vi "Coincident panel edges test.vi"(1 "epsilon":sgl, 3 "V1_1":sgl[](array[numeric])=[1.0, 0.0, 0.0], 4 "V1_0":sgl[](array[numeric])=[1.0, 0.0, 0.0], 5 "V0_1":sgl[](array[numeric])=[1.0, 0.0, 0.0], 6 "V0_0":sgl[](array[numeric])=[1.0, 0.0, 0.0]) -> (0 "Edges are coincident":bool)   [LabVIEW 2017]
panel:
  # "PN 23/10/17"
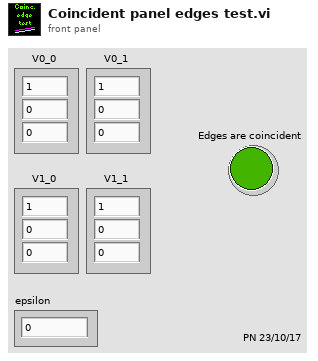
[diagram p1: front panel]
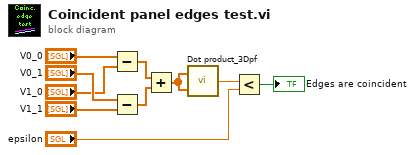
[diagram p0: block diagram]
diagram:
  n1 = Subtract(x="V0_0", y="V1_0") -> (x-y=w10:sgl[])
  n2 = Subtract(x="V0_1", y="V1_1") -> (x-y=w9:sgl[])
  n3 = Add(x=w10, y=w9) -> (x+y=w8:sgl[])
  n4 = call "Dot product_3Dpf.vi"("B"=w8, "A"=w8) -> ("A . B"=w7:sgl)
  n5 = Less?(x=w7, y="epsilon") -> (x < y?=→"Edges are coincident":bool)
